vi "SLAM.vi"(8 "error in":errorcluster, 9 "deltaPosition":cluster{"X":dbl, "Y":dbl, "Angle":dbl}, 10 "Walls":T1(array[cluster])) -> (0 "error out":errorcluster, 1 "RobotPosition":cluster{"X":dbl, "Y":dbl, "Angle":dbl}, 2 "Walls out":cluster{"X":dbl, "Y":dbl}[](array[cluster]))   [LabVIEW 2009, in "Main.lvlib"]
doc: "Main SLAM subroutine. Using landmarks, odometry data, finds robot position in the environment."
uses:
  Main.lvlib
  LV_SLAM/LV_SLAM.lvlib
panel:
  out "Xout":dbl[](array[numeric])
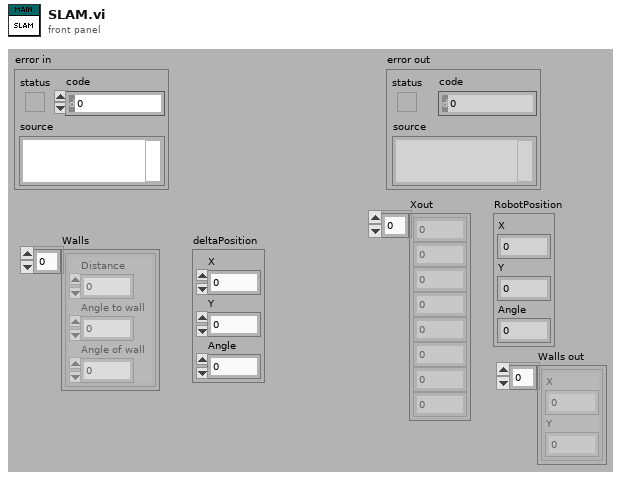
[diagram p1: front panel]
types:
  T1 = cluster{"Distance":dbl, "Angle to wall":dbl, "Angle of wall":dbl}[]
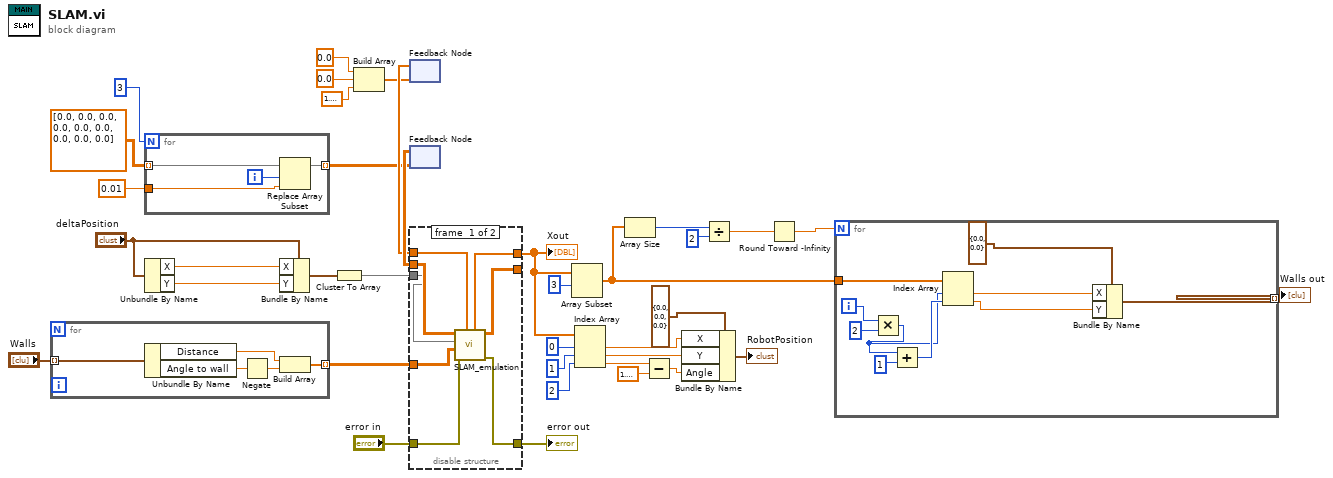
[diagram p0: block diagram]
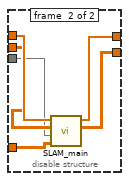
[diagram p2: hidden frame]
diagram:
  n1 = for {
    tunnel: "Walls" -> [w43] mode=indexing
    tunnel: [w41] -> w29 mode=indexing
    n2 = Unbundle By Name(w43) -> ("Distance"=w42:dbl, "Angle to wall"=w39:dbl)
    n3 = Negate(x=w39) -> (-x=w40:dbl)
    n4 = Build Array(w42, w40) -> (w41:dbl[])
  }
  n5 = for {
    N: 3 -> [_]
    tunnel: dbl[][] [[0.0, 0.0, 0.0], [0.0, 0.0, 0.0], [0.0, 0.0, 0.0]] ("Pout") -> [w47] mode=indexing
    tunnel: 0.01 -> [w46]
    tunnel: [w44] -> w32 mode=indexing
    i -> [w45]
    n6 = Replace Array Subset(array=w47, new element=w46, index=w45) -> (w44:dbl[])
  }
  n7 = Unbundle By Name("deltaPosition") -> ("X"=w2:dbl, "Y"=w1:dbl)
  n8 = Bundle By Name(cluster="deltaPosition", "X"=w2, "Y"=w1) -> (w18:cluster{"X":dbl, "Y":dbl, "Angle":dbl})
  n9 = Cluster To Array(cluster=w18) -> (array=w31:dbl[])
  n10 = Build Array(0.0 ("element"), 0.0 ("element"), 1.5707963267948966) -> (w17:dbl[])
  n11 = feedback #1(w17) -> (w36:dbl[])
  n12 = feedback #2(w32) -> (w37:dbl[][])
  n13 = disable-structure shown="Enabled" {
    disable-tunnel: [w52 w58] -> w38
    disable-tunnel: w37 -> [w53 w60]
    disable-tunnel: w36 -> [w55 w61]
    disable-tunnel: w31 -> [w50 w57]
    disable-tunnel: w29 -> [w51 w56]
    disable-tunnel: "error in" -> [w49 _]
    disable-tunnel: [w48 _] -> w27
    disable-tunnel: [w54 w59] -> w10
    frame #0 {
      n14 = call "SLAM_emulation.vi"("X"=w55, "error in"=w49, "measurements"=w51, "dX"=w50, "P"=w53) -> ("error out"=w48:errorcluster, "Pout"=w52:dbl[][], "Xout"=w54:dbl[])  [unwired: 2 in, 2 out]
    }
    frame #1 {
      n15 = call "SLAM_main.vi"("measurements"=w56, "dX"=w57, "P"=w60, "X"=w61) -> ("Pout"=w58:dbl[][], "Xout"=w59:dbl[])  [unwired: 4 in, 2 out]
    }
  }
  "error out" <- w27
  "Xout" <- w10
  n16 = Array Subset(array=w10, index=3) -> (w4:dbl[])  [unwired: 1 in]
  n17 = Index Array(array=w10, index #1=0 ("index"), index #2=1 ("index"), index #3=2 ("index")) -> (element #1=w21:dbl, element #2=w20:dbl, element #3=w12:dbl)
  n18 = Array Size(array=w4) -> (size(s)=w8:i32)
  n19 = Subtract(x=w12, y=1.5707963267948966) -> (x-y=w11:dbl)
  n20 = Bundle By Name(cluster=cluster{"X":dbl, "Y":dbl, "Angle":dbl} {"X"=0.0, "Y"=0.0, "Angle"=0.0} ("RobotPosition 2"), "X"=w21, "Y"=w20, "Angle"=w11) -> (→"RobotPosition":cluster{"X":dbl, "Y":dbl, "Angle":dbl})
  n21 = Divide(x=w8, y=2) -> (x/y=w6:dbl)
  n22 = Round Toward -Infinity(1:w6) -> (0:w5:dbl)
  n23 = for {
    N: w5 -> [_]
    tunnel: w4 -> [w71]
    tunnel: [w67] -> w3 mode=indexing
    i -> [w64]
    n24 = Multiply(x=w64, y=2) -> (x*y=w63:i32)
    n25 = Add(x=w63, y=1) -> (x+y=w69:i32)
    n26 = Index Array(array=w71, index #1=w63, index #2=w69) -> (element #1=w66:dbl, element #2=w65:dbl)
    n27 = Bundle By Name(cluster=cluster{"X":dbl, "Y":dbl} {"X"=0.0, "Y"=0.0} ("Wall"), "X"=w66, "Y"=w65) -> (w67:cluster{"X":dbl, "Y":dbl})
  }
  "Walls out" <- w3
